vi "Swap DDS and CS.vi"(6 "Variant in":variant, 7 "Shift Pressed?":bool, 8 "error in (no error)":errorcluster, 10 "QD Combo Box Ref":refnum<vi>, 11 "QD Launch VI Ref":refnum<vi>) -> (0 "error out":errorcluster, 4 "Variant out":variant)   [LabVIEW 2017]
doc: "This VI checks selected node and either replaces Case Structure with Diagram Disable Structure, or Disable Structure with Case Structure. \nSuggestions from this comment were applied: https://forums.ni.com/t5/LabVIEW-Idea-Exchange/Add-the-ability-to-replace-a-disable-structure-with-a-case/idi-p/1322855/page/2?profile.language=en#comments \n\nDefault Shortcut - [Y]"
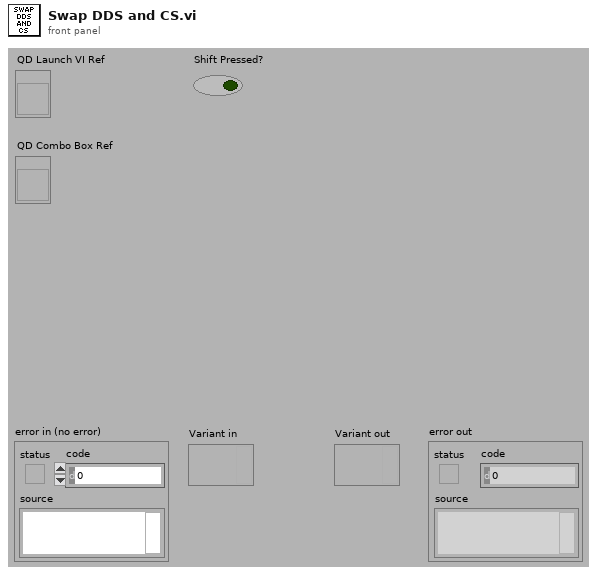
[diagram p1: front panel]
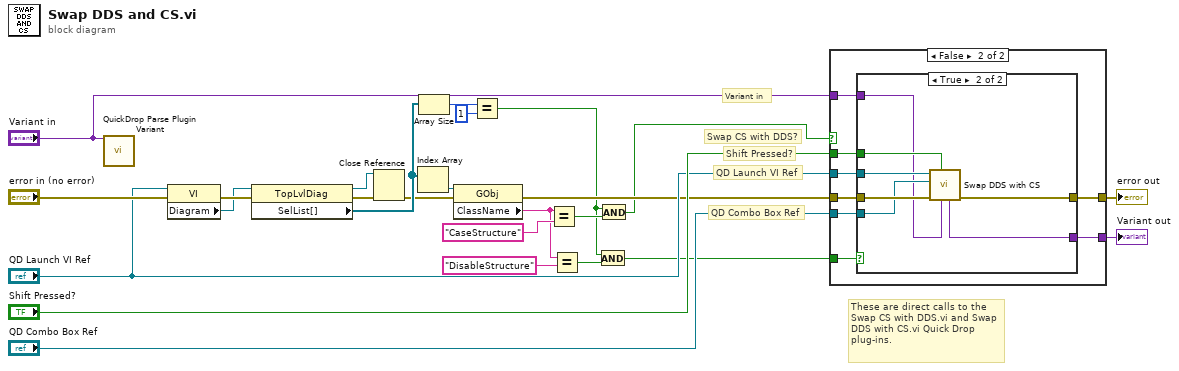
[diagram p0: block diagram]
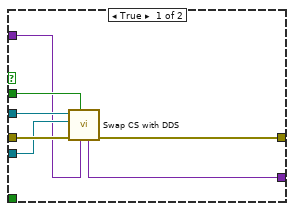
[diagram p2: hidden frame]
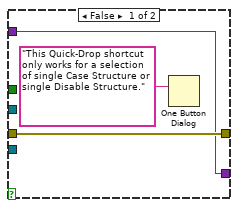
[diagram p3: hidden frame]
diagram:
  # "Swap CS with DDS?"
  # "Variant in"
  # "Shift Pressed?"
  # "QD Launch VI Ref"
  # "QD Combo Box Ref"
  # "These are direct calls to the Swap CS with DDS.vi and Swap DDS with CS.vi Quick Drop plug-ins."
  n1 = call <vilib>:"QuickDrop Parse Plugin Variant.vi"("QDKS Variant in"="Variant in") -> ()  [unwired: 12 in, 3 out]
  n2 = property class="VI"(reference="QD Launch VI Ref", error in="error in (no error)") -> (error out=w18:errorcluster, "Diagram"=w17:refnum<vi>)  [unwired: 1 out]
  n3 = property class="TopLvlDiag"(reference=w17, error in=w18) -> (reference out=w15:refnum<vi>, error out=w16:errorcluster, "SelList[]"=w10:refnum<vi>[])
  n4 = Close Reference(reference=w15, error in (no error)=w16) -> (error out=w8:errorcluster)
  n5 = Index Array(array=w10) -> (element=w14:refnum<vi>)  [unwired: 1 in]
  n6 = Array Size(array=w10) -> (size(s)=w12:i32)
  n7 = property class="GObj"(reference=w14, error in=w8) -> (error out=w9:errorcluster, "ClassName"=w5:string)  [unwired: 1 out]
  n8 = Equal?(x=w12, y=1) -> (x = y?=w2:bool)
  n9 = Equal?(x=w5, y="CaseStructure") -> (x = y?=w6:bool)
  n10 = Equal?(x=w5, y="DisableStructure") -> (x = y?=w3:bool)
  n11 = And(x=w2, y=w3) -> (x .and. y?=w1:bool)
  n12 = And(x=w2, y=w6) -> (x .and. y?=w7:bool)
  n13 = case shown="False" w7 {
    tunnel: w9 -> [w32 w40]
    tunnel: [w31 w39] -> w24
    tunnel: "Variant in" -> [w26 w34]
    tunnel: "Shift Pressed?" -> [w30 w38]
    tunnel: "QD Launch VI Ref" -> [w29 w37]
    tunnel: "QD Combo Box Ref" -> [w28 w36]
    tunnel: [w27 w35] -> w19
    tunnel: w1 -> [_ w33]
    frame True {
      n14 = call "Swap CS with DDS.vi"("Variant in"=w26, "Shift Pressed?"=w30, "error in (no error)"=w32, "QD Combo Box Ref"=w28, "QD Launch VI Ref"=w29) -> ("error out"=w31:errorcluster, "Variant out"=w27:variant)  [unwired: 5 in]
    }
    frame False {
      n15 = case shown="True" w33 {
        tunnel: w40 -> [w43 w50]
        tunnel: [w43 w49] -> w39
        tunnel: w38 -> [_ w48]
        tunnel: w37 -> [_ w47]
        tunnel: w36 -> [_ w46]
        tunnel: [w42 w45] -> w35
        tunnel: w34 -> [w42 w44]
        frame False {
          n16 = One Button Dialog(message="This Quick-Drop shortcut only works for a selection of single Case Structure or single Disable Structure.") -> ()  [unwired: 1 in, 1 out]
        }
        frame True {
          n17 = call "Swap DDS with CS.vi"("Variant in"=w44, "Shift Pressed?"=w48, "error in (no error)"=w50, "QD Combo Box Ref"=w46, "QD Launch VI Ref"=w47) -> ("error out"=w49:errorcluster, "Variant out"=w45:variant)  [unwired: 5 in]
        }
      }
    }
  }
  "error out" <- w24
  "Variant out" <- w19
